vi "String_Wait.vi"(11 "String":string="Wait for Temperature, Timeout 300sec, Continue") -> (0 "On timeout":i32(ring) items=["Continue", "Abort "], 1 "Timeout(s)":i16=300, 2 "Field":bool caption="Wait magnetic field stable", 3 "Temperature":bool=TRUE caption="Wait temperature stable")   [LabVIEW 2017]
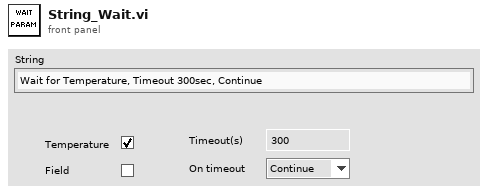
[diagram p1: front panel]
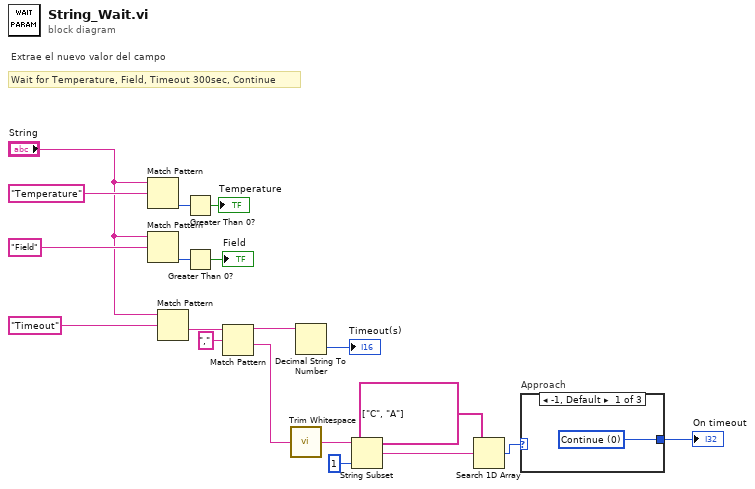
[diagram p0: block diagram]
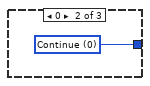
[diagram p2: hidden frame]
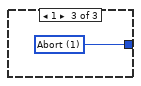
[diagram p3: hidden frame]
diagram:
  # "Wait for Temperature, Field, Timeout 300sec, Continue"
  # "Extrae el nuevo valor del campo"
  n1 = Match Pattern(string="String", regular expression="Temperature") -> (offset past match=w13:i32)  [unwired: 1 in, 3 out]
  n2 = Match Pattern(string="String", regular expression="Field") -> (offset past match=w11:i32)  [unwired: 1 in, 3 out]
  n3 = Match Pattern(string="String", regular expression="Timeout") -> (after substring=w7:string)  [unwired: 1 in, 3 out]
  n4 = Greater Than 0?(x=w13) -> (x > 0?=→"Temperature":bool)
  n5 = Greater Than 0?(x=w11) -> (x > 0?=→"Field":bool)
  n6 = Match Pattern(string=w7, regular expression=",") -> (before substring=w2:string, after substring=w3:string)  [unwired: 1 in, 2 out]
  n7 = call <vilib>:"Trim Whitespace.vi"("string"=w3) -> ("trimmed string"=w15:string)  [unwired: 1 in]
  n8 = Decimal String To Number(string=w2) -> (number=→"Timeout(s)":i32)  [unwired: 2 in, 1 out]
  n9 = String Subset(string=w15, length (rest)=1 ("length (rest)")) -> (substring=w18:string)  [unwired: 1 in]
  n10 = Search 1D Array(1D array=string[] ["C", "A"], element=w18) -> (index of element=w19:i32)  [unwired: 1 in]
  n11 = case "Approach" shown="-1, Default" w19 {
    tunnel: [w20 w21 w22] -> w4
    frame -1, Default {
      w20 = 0 items=["Continue", "Abort "] ("On timeout")
    }
    frame 0 {
      w21 = 0 items=["Continue", "Abort "] ("On timeout")
    }
    frame 1 {
      w22 = 1 items=["Continue", "Abort "] ("On timeout")
    }
  }
  "On timeout" <- w4
